vi "Stream Circle (FW7).vi"(4 "Direction (0: clockwise)":u16(ring) items=["clockwise", "counter-clockwise"], 6 "Position Mode (0: absolute)":u16(ring) items=["absolute", "relative"], 7 "Center":i64[](array[numeric]), 8 "error in (no error)":errorcluster, 9 "Device Number":string, 10 "Stream Number (1)":u8=1, 11 "VISA resource name":refnum<visa-resource-name>) -> (0 "error out":errorcluster, 3 "VISA resource name out":refnum<visa-resource-name>)   [LabVIEW 2015, in "Zaber A Series.lvlib"]
doc: "Adds a circle command to an open stream. The position where the previous stream command leaves the device will be a point on the circle. The Center Position input specifies where the center of the circle will be, either in absolute coordinates or relative to the device position; the Position Mode input controls whether it is absolute or relative.\n\nThe center point is specified in microstep units - use the Convert Position to Device Units VI to convert from standard measurements.\n\nThis VI does not check in advance for error conditions such as streams not being supported or the stream not being open.\n\nThis VI requires that the Initialize VI has been called with the same serial port and that the specified stream is open."
uses:
  Zaber A Series.lvlib
  Private/All Commands.ctl
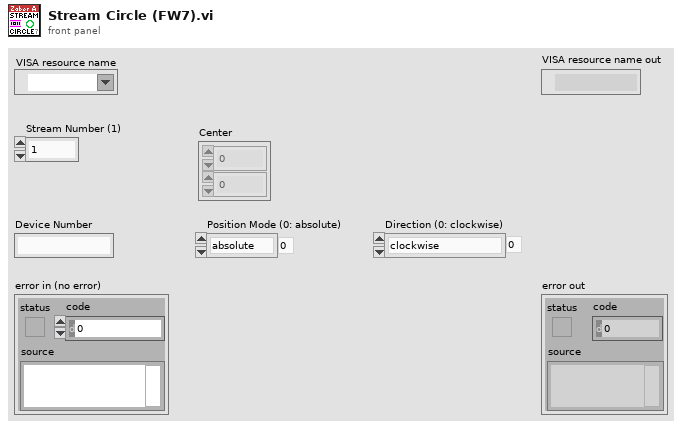
[diagram p1: front panel]
types:
  T1 = typedef "Zaber A Series.lvlib/All Commands.ctl" = string
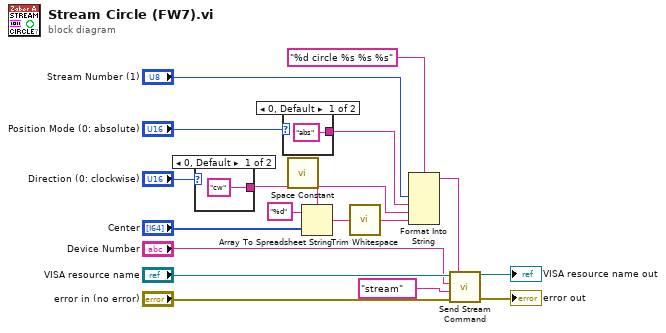
[diagram p0: block diagram]
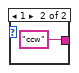
[diagram p2: hidden frame]
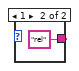
[diagram p3: hidden frame]
diagram:
  n1 = case shown="0, Default" "Direction (0: clockwise)" {
    tunnel: ["cw" "ccw"] -> w5
    frame 0, Default {
    }
    frame 1 {
    }
  }
  n2 = case shown="0, Default" "Position Mode (0: absolute)" {
    tunnel: ["abs" "rel"] -> w6
    frame 0, Default {
    }
    frame 1 {
    }
  }
  n3 = call <vilib>:"Space Constant.vi"() -> ("String"=w3:string)
  n4 = Array To Spreadsheet String(delimiter (Tab)=w3, array="Center", 3:"%d" ("format string")) -> (spreadsheet string=w9:string)
  n5 = call <vilib>:"Trim Whitespace.vi"("string"=w9) -> ("trimmed string"=w4:string)  [unwired: 1 in]
  n6 = Format Into String(format string="%d circle %s %s %s", "Stream Number (1)", w6, w5, w4) -> (resulting string=w2:string)  [unwired: 2 in, 1 out]
  n7 = call "Send Stream Command.vi"("Data"=w2, "error in (no error)"="error in (no error)", "Command"=T1 "stream" ("Complete Command List"), "Device Number"="Device Number", "VISA resource name"="VISA resource name") -> ("error out"=→"error out":errorcluster, "VISA resource name out"=→"VISA resource name out":refnum<visa-resource-name>)  [unwired: 5 in]
